vi "Host-Top-Level.vi"() -> ()   [LabVIEW 2017]
uses:
  State.ctl
  <vilib>/FPGAPlugInAG/PXIe-6592R/niLvFpga_Open_PXIe-6592R.vi
  <vilib>/rvi/interface/common/dynamic/niFpgaDynamicAddResources.vi
  <vilib>/Utility/error.llb/Error Cluster From Error Code.vi
  <vilib>/rvi/errors/niLvFpgaAdjustHostInterfaceError.vi
  <vilib>/FPGAPlugInAG/Dynamic/niLvFpga_Close_Dynamic.vi
  <vilib>/rvi/interface/nirviOpenFPGA/nirviOpenFPGA.xnode
  FPGA Bitfiles/02MicroBlazeMcsI_FPGATarget_Fpga-6592-Top-Le_1BKGQ3Zm+NY.lvbitx
  Fpga-6592/Fpga-6592-Top-Level.vi
  <vilib>/rvi/interface/nirviReadWriteControl/nirviReadWriteControl.xnode
  <vilib>/rvi/interface/nirviMethod/nirviMethod.xnode
  <vilib>/rvi/interface/nirviCloseFPGA/nirviCloseFPGA.xnode
  <vilib>/rvi/errors/niLvFpgaMergeErrorWithErrorCode.vi
  <vilib>/FPGAPlugInAG/Dynamic/niLvFpga_ReadFifo_Dynamic.vi
  NiFpgaLv.dll
  <vilib>/rvi/interface/Simulation/niFpgaSimulationCallBeginRW.vi
  <vilib>/FPGAPlugInAG/Dynamic/niLvFpga_WriteFifo_Dynamic.vi
panel:
  out "error out":errorcluster
  out "addr_strobe_count":u16
  out "write_strobe_count":u16
  out "read_strobe_count":u16
  out "GPO 1":u32
  out "GPO 3":u32
  out "GPO 2":u32
  in  "Read all GPO":bool
  out "GPO_2":u32
  in  "GPI_1":u32
  in  "Test GPIO Write-Read":bool
  in  "Interrupt Number":fxp<+,4,4>=1.0
  out "Read Data":u32[](array[numeric]) format="%.0x"
  in  "DataToSend":u32[](array[numeric])=[240, 241, 242, 243, 244, 245] format="%.0x"
  in  "Send":bool
  in  "Stop":bool
  in  "error in":errorcluster
  # "Send a packet of data, read the same data\necho'd back by MicroBlaze MCS"
  # "GPO 2 = GPI 1 * 2"
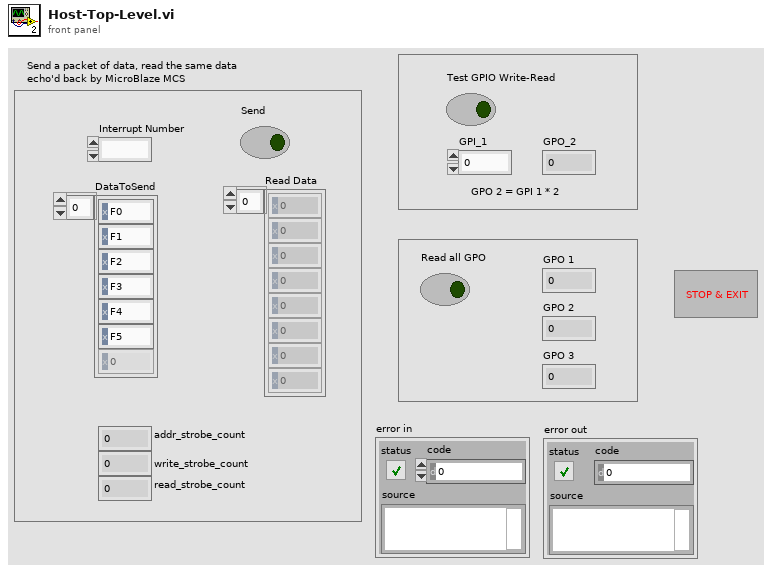
[diagram p1: front panel]
types:
  T1 = typedef "State.ctl" = enum16{"Initialize", "Idle", "Read", "Exit"}
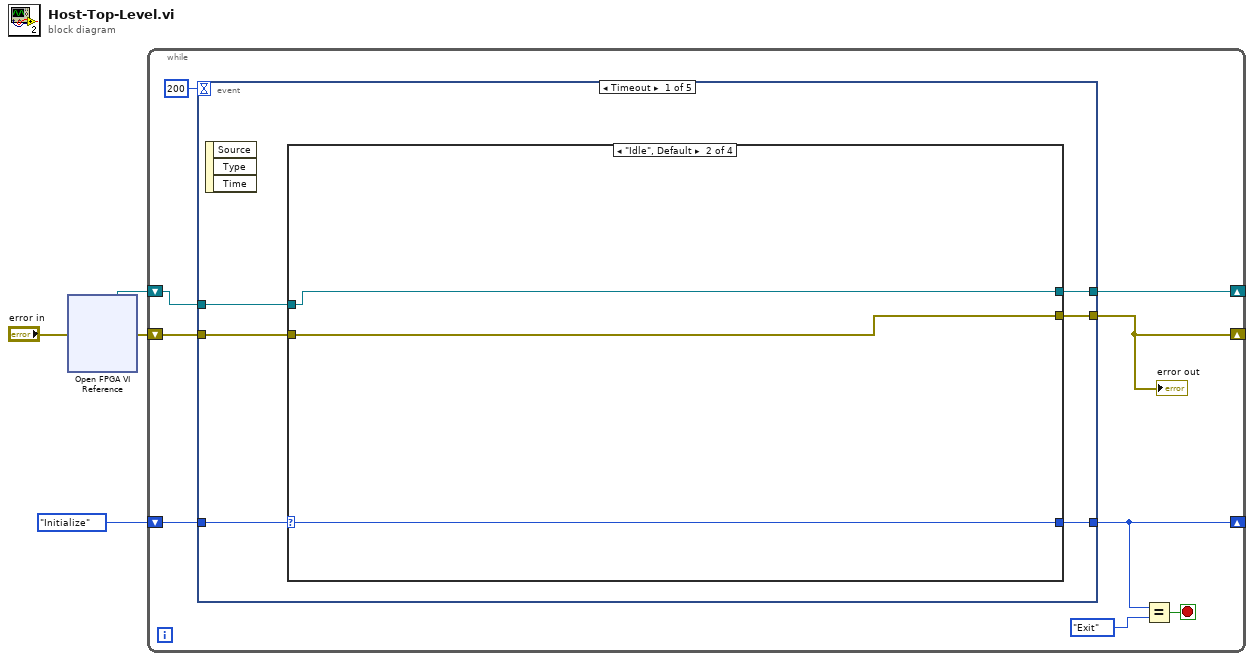
[diagram p0: block diagram]
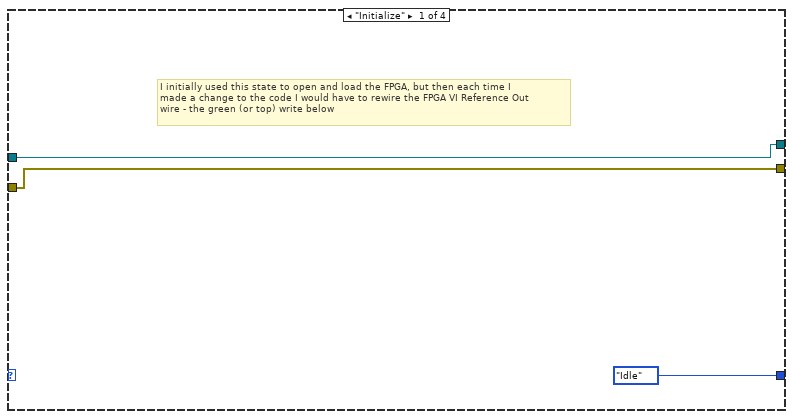
[diagram p2: hidden frame]
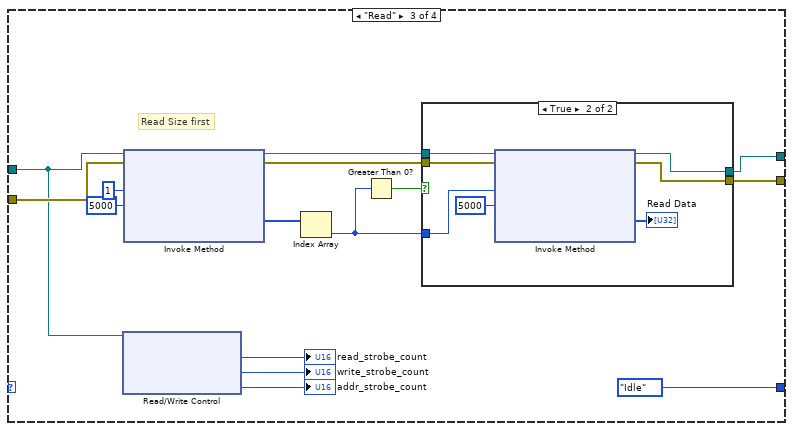
[diagram p3: hidden frame]
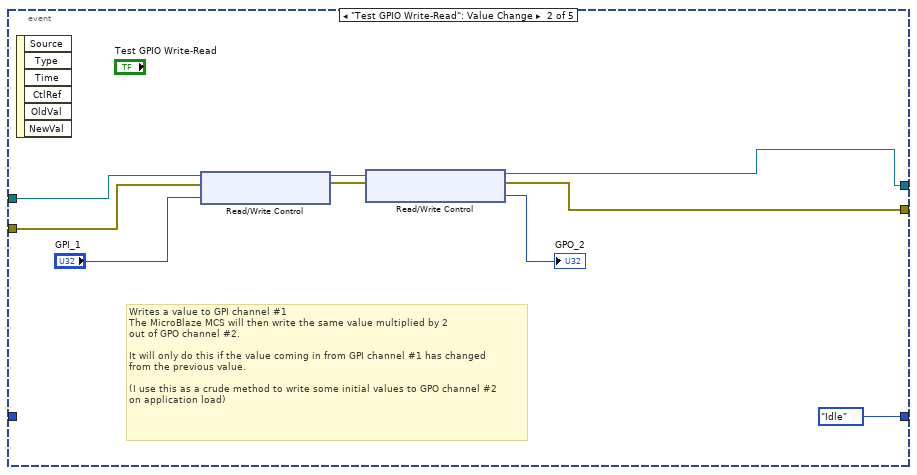
[diagram p6: hidden frame]
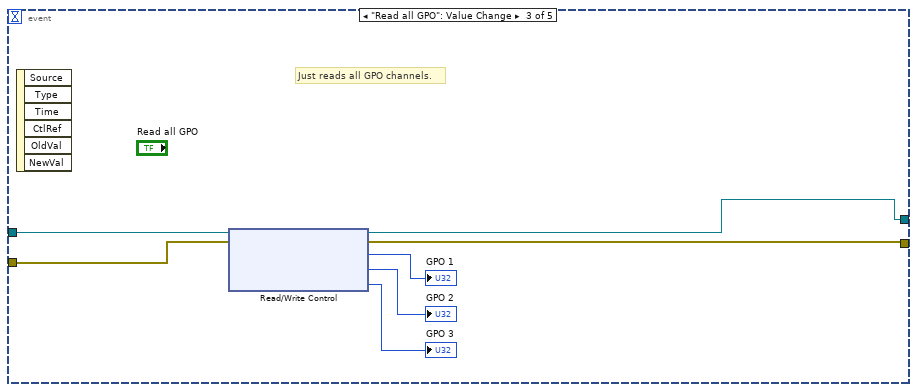
[diagram p7: hidden frame]
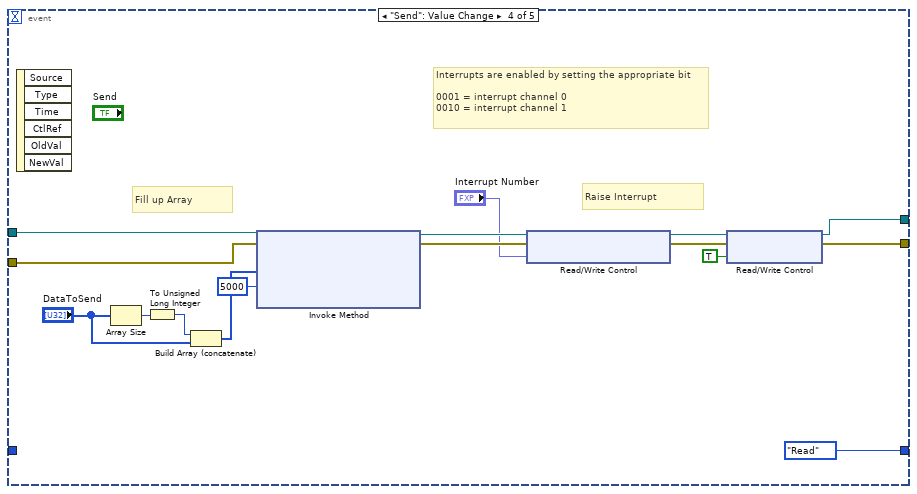
[diagram p8: hidden frame]
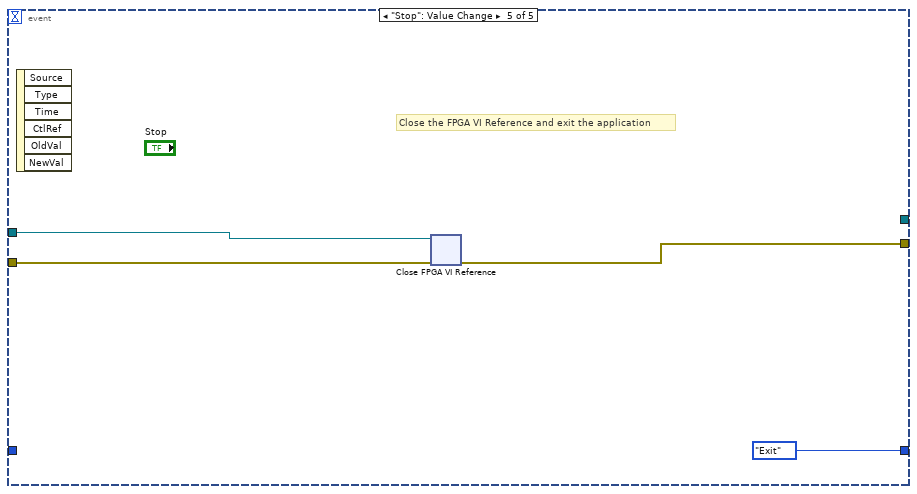
[diagram p9: hidden frame]
diagram:
  n1 = xnode "Open FPGA VI Reference"("error in"="error in") -> ("FPGA VI Reference Out"=w3:refnum<k20>, "error out"=w1:errorcluster)  [unwired: 1 in]
  n2 = while {
    shift-right: [w7] -> _
    shift-left: State."Initialize" ("Enum") -> [w13]
    shift-right: [w8] -> _
    shift-left: w1 -> [w9]
    shift-right: [w6] -> _
    shift-left: w3 -> [w5]
    stop <- w11 stop-if-true
    n3 = event shown="[0] Timeout" {
      selector: _ -> [_ _ _ _ _]
      dyn-events: _ -> [_ _ _ _ _]
      timeout: 200 -> [_ _ _ _ _]
      tunnel: [w17 State."Idle" ("Enum") _ State."Read" ("Enum") State."Exit" ("Enum")] -> w7
      tunnel: w13 -> [w16 _ _ _ _]
      tunnel: w5 -> [w15 w60 w68 w82 w86]
      tunnel: w9 -> [w19 w59 w67 w81 w85]
      tunnel: [w18 w55 w66 w80 w84] -> w8
      tunnel: [w14 w53 w62 w69 _] -> w6
      event Timeout {
        n4 = event-data() -> ()  [unwired: 1 in, 3 out]
        n5 = case shown="\"Idle\", Default" w16 {
          selector: w16 -> [_ w24 _ w51]
          tunnel: w19 -> [w21 w25 w40 w52]
          tunnel: [w21 w25 w34 w52] -> w18
          tunnel: w15 -> [w20 w23 w30 w50]
          tunnel: [State."Idle" ("Enum") w24 State."Idle" ("Enum") w51] -> w17
          tunnel: [w20 w23 w29 w50] -> w14
          frame "Initialize" {
            # "I initially used this state to open and load the FPGA, but then each time I \nmade a change to the code I would have to rewire the FPGA VI Reference Out \nwire - the green (or top) write below"
          }
          frame "Idle", Default {
          }
          frame "Read" {
            # "Read Size first"
            n6 = xnode "Read/Write Control"("FPGA VI Reference In"=w30) -> ("read_strobe_count"=→"read_strobe_count":u16, "write_strobe_count"=→"write_strobe_count":u16, "addr_strobe_count"=→"addr_strobe_count":u16)  [unwired: 1 in, 2 out]
            n7 = xnode "Invoke Method"("FPGA VI Reference In"=w30, "error in"=w40, "Number of Elements"=u32 1, "Timeout (ms)"=5000) -> ("FPGA VI Reference Out"=w36:refnum<k20>, "error out"=w37:errorcluster, "Data"=w35:u32[])  [unwired: 1 out]
            n8 = Index Array(array=w35) -> (element=w32:u32)  [unwired: 1 in]
            n9 = Greater Than 0?(x=w32) -> (x > 0?=w31:bool)
            n10 = case shown="True" w31 {
              tunnel: w37 -> [w42 w49]
              tunnel: w36 -> [w41 w48]
              tunnel: [w42 w46] -> w34
              tunnel: [w41 w45] -> w29
              tunnel: w32 -> [_ w43]
              frame False {
              }
              frame True {
                n11 = xnode "Invoke Method"("FPGA VI Reference In"=w48, "error in"=w49, "Number of Elements"=w43, "Timeout (ms)"=5000) -> ("FPGA VI Reference Out"=w45:refnum<k20>, "error out"=w46:errorcluster, "Data"=→"Read Data":u32[])  [unwired: 1 out]
              }
            }
          }
          frame "Exit" {
          }
        }
      }
      event "Test GPIO Write-Read": Value Change {
        # "Writes a value to GPI channel #1\nThe MicroBlaze MCS will then write the same value multiplied by 2\nout of GPO channel #2.\n\nIt will only do this if the value coming in from GPI channel #1 has changed\nfrom the previous value.\n\n(I use this as a crude method to write some initial values to GPO channel #2\non application load)"
        n12 = event-data() -> ()  [unwired: 1 in, 6 out]
        n13 = xnode "Read/Write Control"("FPGA VI Reference In"=w60, "error in"=w59, "d_mcs_i\\gpio_rtl_tri_i"="GPI_1") -> ("FPGA VI Reference Out"=w54:refnum<k20>, "error out"=w57:errorcluster)
        n14 = xnode "Read/Write Control"("FPGA VI Reference In"=w54, "error in"=w57) -> ("FPGA VI Reference Out"=w53:refnum<k20>, "error out"=w55:errorcluster, "d_mcs_i\\gpio2_rtl_tri_o"=→"GPO_2":u32)
      }
      event "Read all GPO": Value Change {
        # "Just reads all GPO channels."
        n15 = event-data() -> ()  [unwired: 1 in, 6 out]
        n16 = xnode "Read/Write Control"("FPGA VI Reference In"=w68, "error in"=w67) -> ("FPGA VI Reference Out"=w62:refnum<k20>, "error out"=w66:errorcluster, "d_mcs_i\\gpio1_rtl_tri_o"=→"GPO 1":u32, "d_mcs_i\\gpio2_rtl_tri_o"=→"GPO 2":u32, "d_mcs_i\\gpio3_rtl_tri_o"=→"GPO 3":u32)
      }
      event "Send": Value Change {
        # "Interrupts are enabled by setting the appropriate bit\n\n0001 = interrupt channel 0\n0010 = interrupt channel 1"
        # "Raise Interrupt"
        # "Fill up Array"
        n17 = event-data() -> ()  [unwired: 1 in, 6 out]
        n18 = Array Size(array="DataToSend") -> (size(s)=w78:i32)
        n19 = To Unsigned Long Integer(number=w78) -> (unsigned 32bit integer=w75:u32)
        n20 = Build Array (concatenate)(w75, "DataToSend") -> (w76:u32[])
        n21 = xnode "Invoke Method"("FPGA VI Reference In"=w82, "error in"=w81, "Data"=w76, "Timeout (ms)"=5000) -> ("FPGA VI Reference Out"=w79:refnum<k20>, "error out"=w80:errorcluster)  [unwired: 1 out]
        n22 = xnode "Read/Write Control"("FPGA VI Reference In"=w79, "d_mcs_i\\INTC_Interrupt"="Interrupt Number") -> ("FPGA VI Reference Out"=w72:refnum<k20>)  [unwired: 1 in, 1 out]
        n23 = xnode "Read/Write Control"("FPGA VI Reference In"=w72, "Write Interrupt"=TRUE) -> ("FPGA VI Reference Out"=w69:refnum<k20>)  [unwired: 1 in, 1 out]
      }
      event "Stop": Value Change {
        # "Close the FPGA VI Reference and exit the application"
        n24 = event-data() -> ()  [unwired: 1 in, 6 out]
        n25 = xnode "Close FPGA VI Reference"("FPGA VI Reference In"=w86, "error in"=w85) -> ("error out"=w84:errorcluster)
      }
    }
    "error out" <- w8
    n26 = Equal?(x=w7, y=State."Exit") -> (x = y?=w11:bool)
  }
